vi "sequence util_error check.vi"(10 "Item Names IN":string[](array[string])=["----------    AH Bridge: Save GPIB address   ", "Write to VISA, GPIB::27::INSTR, FILE STORE GPIB USERPON", "----------    LakeShore 340 controller: change heater power (0-5, 0: off)  ", "Write to VISA, GPIB::12::INSTR, RANGE 0", "----------    Scheduled T-control for the He3 system   ", "Wait for 12 hour", "Set Temperature LS336 ( GPIB0::12::INSTR ) 45 K at 0 K/min, Output 1", "Wait for 60 s", "Wait for Temperature Less than 1.8 K Sensor C of LS336 ( GPIB0::14::INSTR ) Timeout 30 min", "Wait for 60 min", "Set Temperature LS336 ( GPIB0::12::INSTR ) 0.1 K at 0 K/min, Output 1", "----------    Motor control (use Instrumet:Set:MotorControl command structure)  ", "Set MotorControl ( BLM ) 12345 0.2", "Wait for VI value localhost, BLM_ManualControl.vi, BLM Position, Within, 12345, 10 min", "Wait for 10 s", "END SEQUENCE"]) -> (2 "indexed Item Names out":string[](array[string]), 3 "error":bool caption="error indicator")   [LabVIEW 2020]
panel:
  in  "Close Window":bool
  in  "sequence in":i32(listbox)
  in  "error in":errorcluster
  out "error out":errorcluster
  # "(can be edited for root commands (commands not in the subsequence))"
  # "`"
  # "If expand macro is ON, sequences are labelled #.n (n= 0 for main command, n>0 for expanded command)."
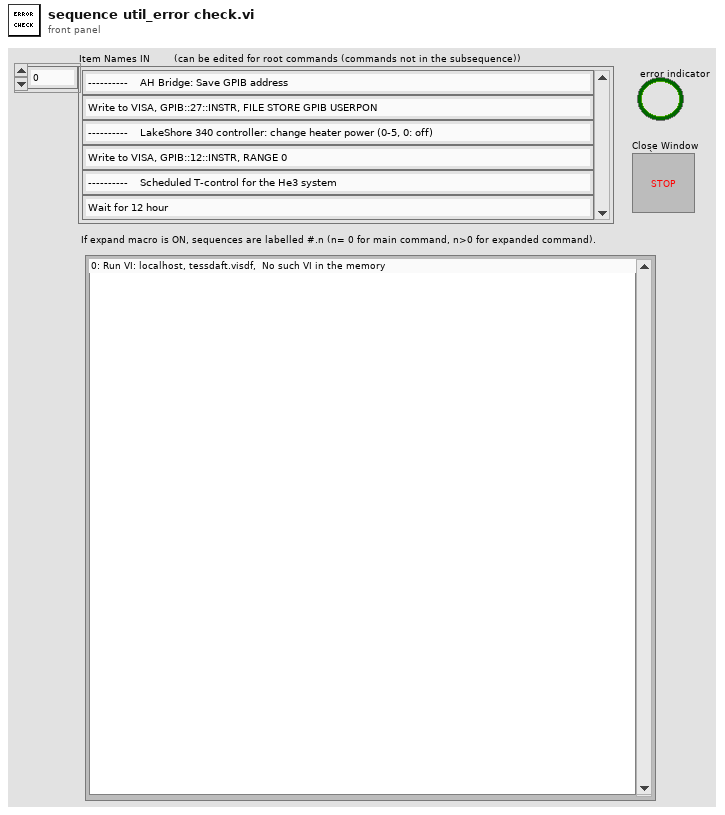
[diagram p1: front panel]
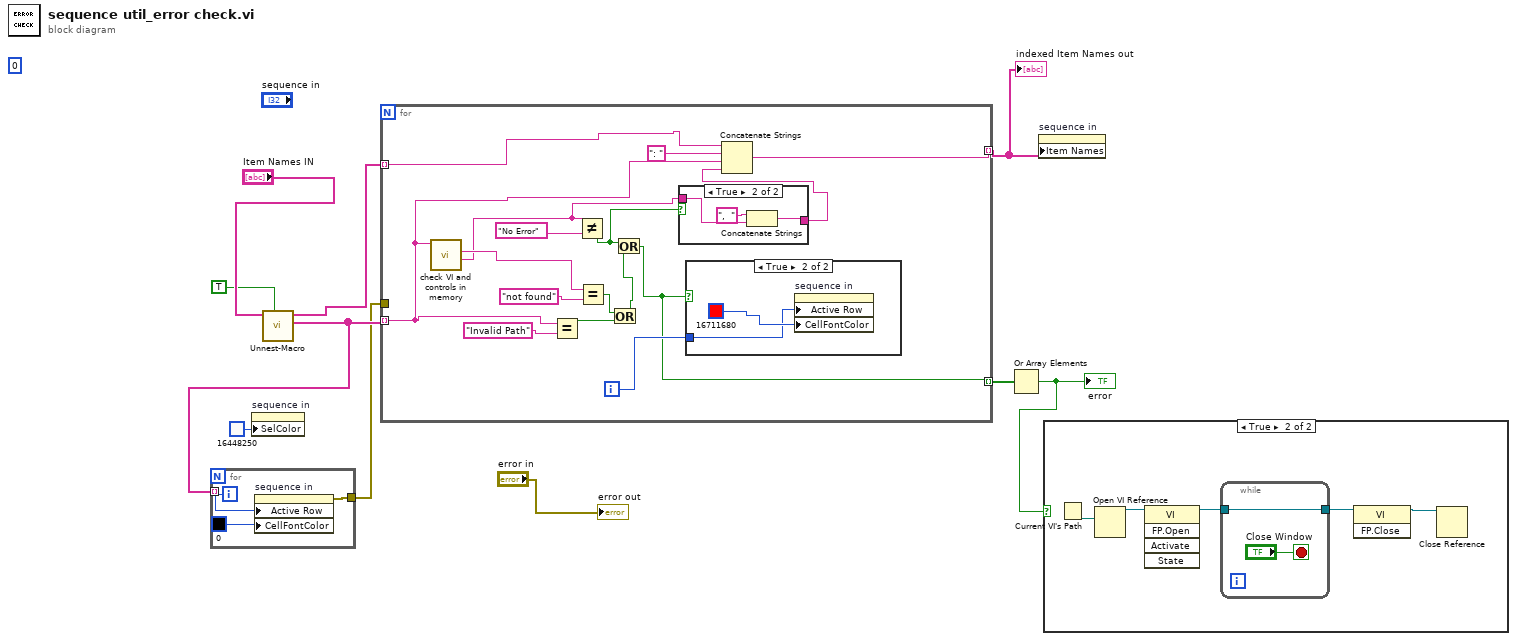
[diagram p0: block diagram]
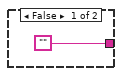
[diagram p3: hidden frame]
diagram:
  (unwired) 0 ("sequence in")
  n1 = property on="sequence in" class="LstBox (strict)"("SelColor"=u32 16448250 ("Selection Color")) -> ()  [unwired: 2 in, 2 out]
  n2 = call "Unnest-Macro.vi"("expand"=TRUE, "Item Names IN"="Item Names IN") -> ("unnested items"=w6:string[], "item index"=w7:string[])  [unwired: 8 in]
  n3 = for {
    tunnel: w6 -> [_] mode=indexing
    tunnel: [w11] -> w5
    i -> [w13]
    n4 = property on="sequence in" class="LstBox (strict)"("Active Row"=w13, "CellFontColor"=u32 0 ("Active Row:Cell Font:Color")) -> (error out=w11:errorcluster)  [unwired: 2 in, 1 out]
  }
  n5 = for {
    tunnel: w6 -> [w21] mode=indexing
    tunnel: [w26] -> w2 mode=indexing
    tunnel: w7 -> [w28] mode=indexing
    tunnel: w5 -> [_]
    tunnel: [w14] -> w3 mode=indexing
    i -> [w25]
    n6 = call "check VI and controls in memory.vi"("Input command"=w21) -> ("error message"=w15:string, "Identifield command"=w20:string)  [unwired: 7 in, 2 out]
    n7 = Equal?(x=w21, y="Invalid Path") -> (x = y?=w22:bool)
    n8 = Not Equal?(x=w15, y="No Error") -> (x != y?=w17:bool)
    n9 = Equal?(x=w20, y="not found") -> (x = y?=w23:bool)
    n10 = Or(x=w23, y=w22) -> (x .or. y?=w18:bool)
    n11 = Or(x=w17, y=w18) -> (x .or. y?=w14:bool)
    n12 = case shown="True" w17 {
      tunnel: ["" w33] -> w16
      tunnel: w15 -> [_ w32]
      frame False {
      }
      frame True {
        n13 = Concatenate Strings(",  " ("string"), w32) -> (w33:string)
      }
    }
    n14 = case shown="True" w14 {
      tunnel: w25 -> [_ w34]
      frame False {
      }
      frame True {
        n15 = property on="sequence in" class="LstBox (strict)"("Active Row"=w34, "CellFontColor"=u32 16711680 ("Active Row:Cell Font:Color")) -> ()  [unwired: 2 in, 2 out]
      }
    }
    n16 = Concatenate Strings(w28, ": ", w21, w16) -> (w26:string)
  }
  "indexed Item Names out" <- w2
  n17 = Or Array Elements(Boolean array=w3) -> (logical OR=w1:bool)
  "error" <- w1
  n18 = property on="sequence in" class="LstBox (strict)"("Item Names"=w2) -> ()  [unwired: 2 in, 2 out]
  n19 = case shown="True" w1 {
    frame False {
    }
    frame True {
      n20 = Current VI's Path() -> (path=w40:path)
      n21 = Open VI Reference(vi path=w40) -> (vi reference=w39:refnum<vi>)  [unwired: 5 in, 1 out]
      n22 = invoke class="VI" method="FP.Open"(reference=w39) -> (reference out=w38:refnum<vi>)  [unwired: 4 in, 4 out]
      n23 = while {
        tunnel: [w41] -> w37
        tunnel: w38 -> [w41]
        stop <- "Close Window" stop-if-true
      }
      n24 = invoke class="VI" method="FP.Close"(reference=w37) -> (reference out=w36:refnum<vi>)  [unwired: 2 in, 2 out]
      n25 = Close Reference(reference=w36) -> ()  [unwired: 1 in, 1 out]
    }
  }
  "error out" <- "error in"
